vi "Actualizar Grafica.vi"(8 "error in (no error)":errorcluster, 11 "Generador de Funciones in":refnum<class "Generador de Funciones.lvclass">=refnum) -> (0 "error out":errorcluster, 3 "Generador de Funciones out":refnum<class "Generador de Funciones.lvclass">)   [LabVIEW 2020, in "Generador de Funciones.lvlib" / "Generador de Funciones.lvclass"]
uses:
  Generador de Funciones.lvclass
  Generador de Funciones.lvclass/Generador de Funciones.ctl
panel:
  in  "Generar Señal":waveform(dbl)
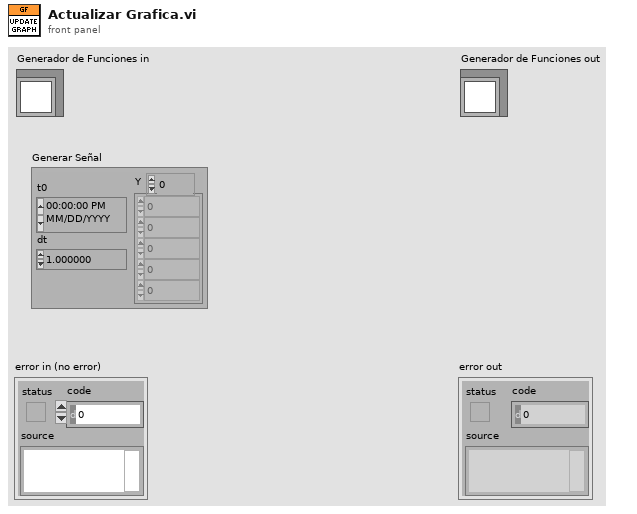
[diagram p1: front panel]
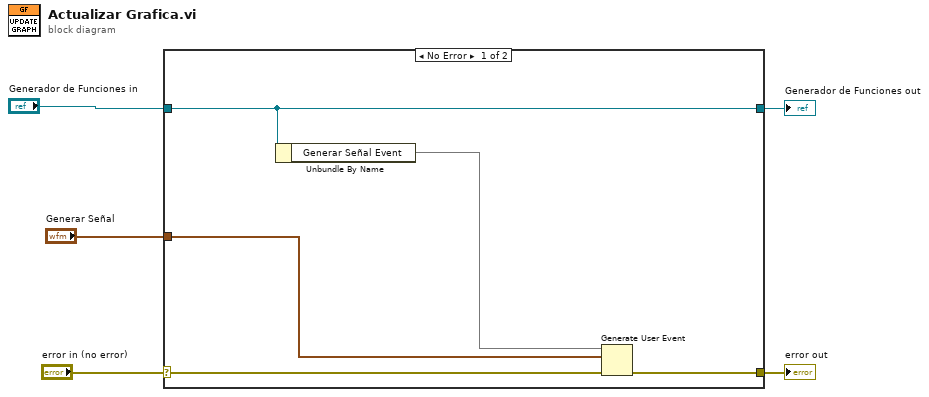
[diagram p0: block diagram]
diagram:
  n1 = case shown="No Error" "error in (no error)" {
    selector: "error in (no error)" -> [w10 w12]
    tunnel: [w8 w12] -> w4
    tunnel: [w9 w11] -> w2
    tunnel: "Generador de Funciones in" -> [w9 w11]
    tunnel: "Generar Señal" -> [w6 _]
    frame No Error {
      n2 = Unbundle By Name(w9) -> ("Generar Señal Event"=w7)
      n3 = Generate User Event(user event=w7, event data cluster=w6, error in=w10) -> (error out=w8:errorcluster)  [unwired: 1 in, 1 out]
    }
    frame Error {
    }
  }
  "error out" <- w4
  "Generador de Funciones out" <- w2
